vi "Battery mcc.vi"() -> ()   [LabVIEW 2021]
panel:
  in  "stop":bool
  out "length":i32
  in  "Array":dbl[](array[numeric])
  out "String":string
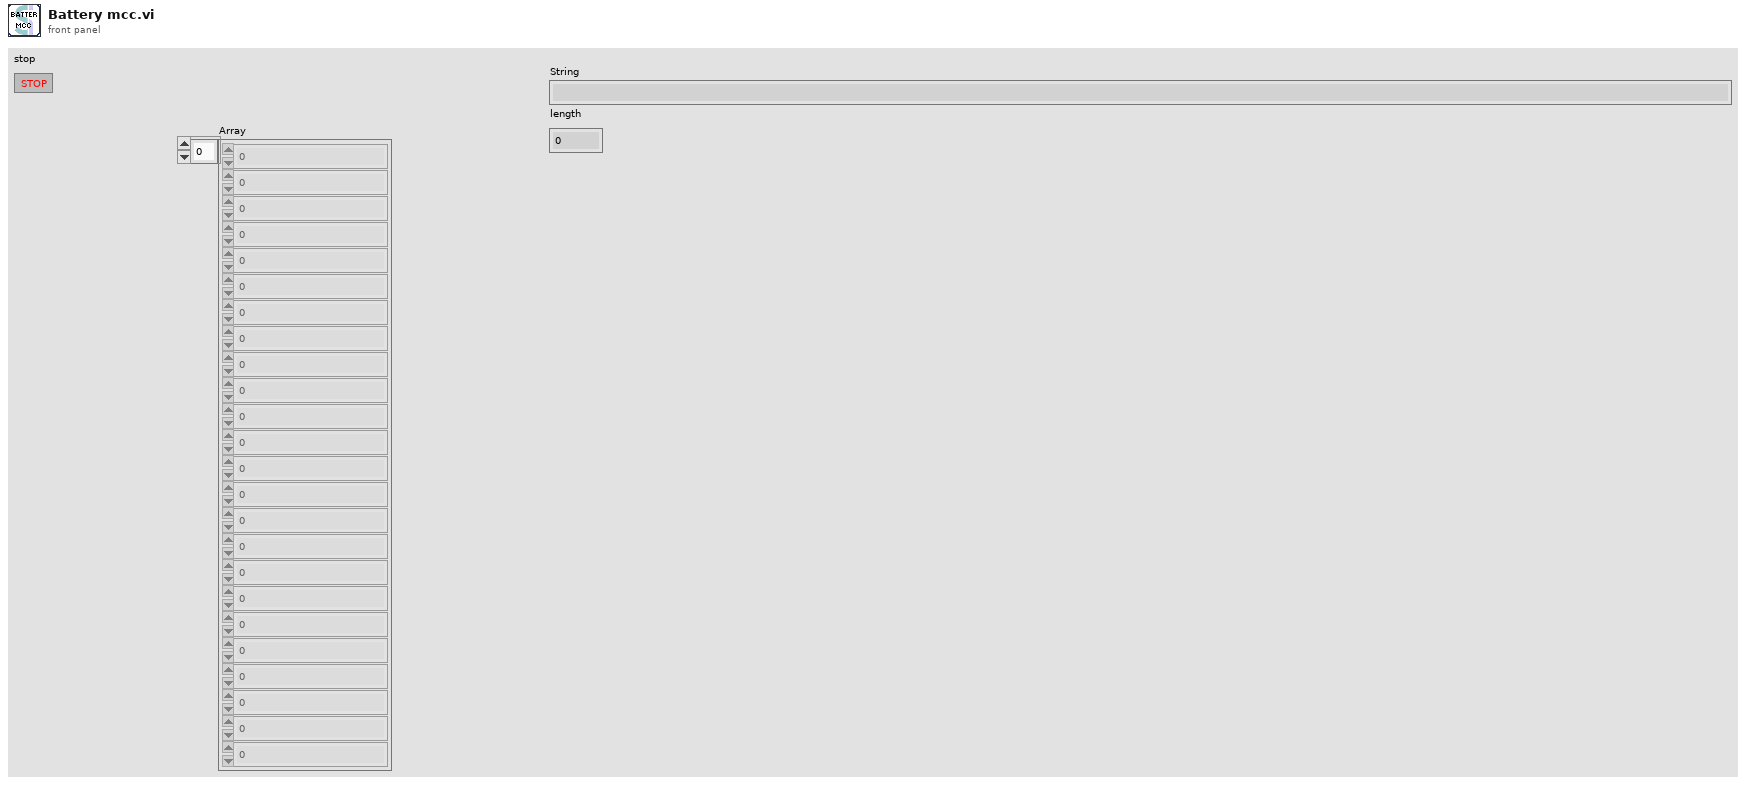
[diagram p1: front panel]
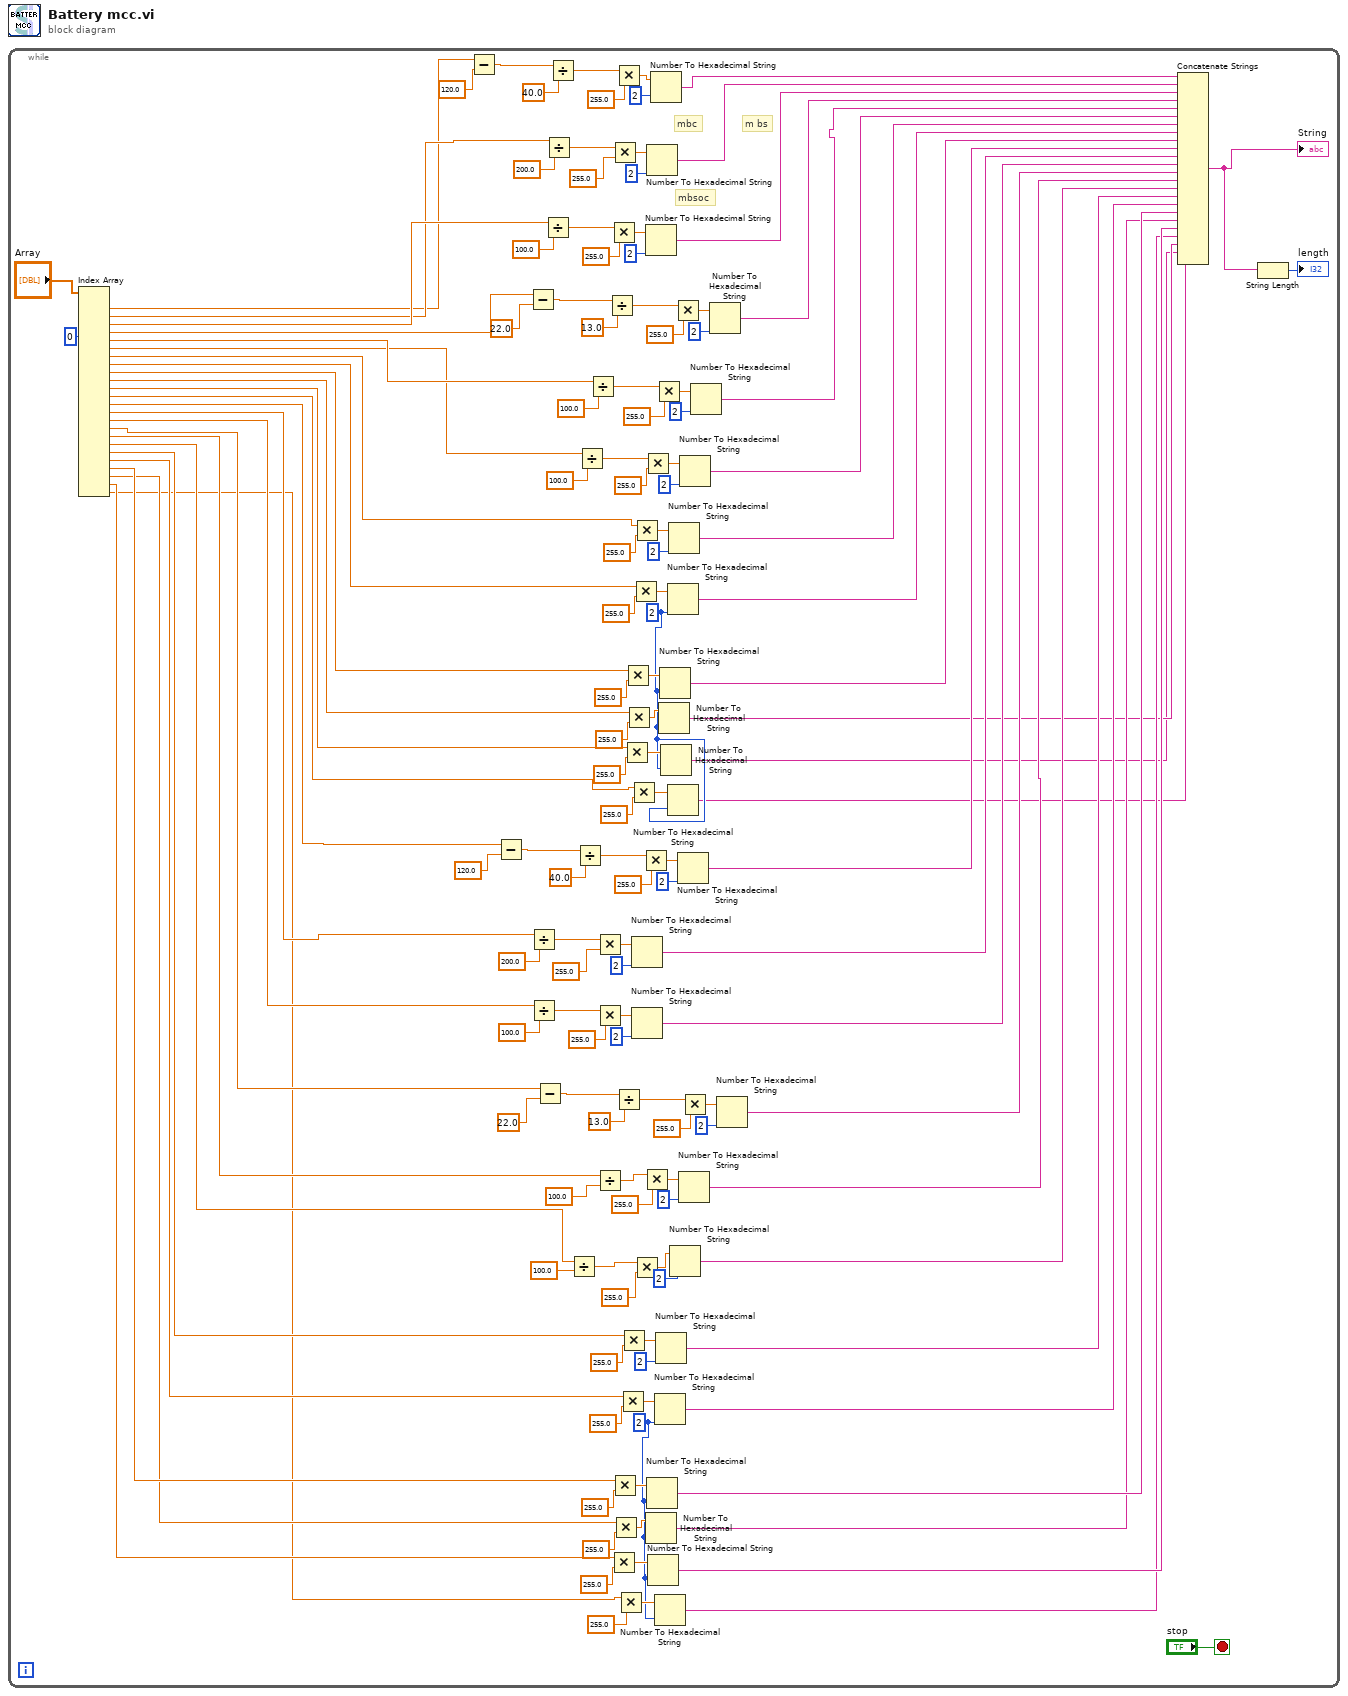
[diagram p0: block diagram]
diagram:
  # "m bs"
  n1 = while {
    stop <- "stop" stop-if-true
    w9 = i16 2 ("width (-)")
    w42 = i16 2 ("width (-)")
    # "mbsoc"
    # "mbc"
    n2 = Index Array(array="Array", index #1=0 ("index")) -> (element #1=w146:dbl, element #2=w147:dbl, element #3=w148:dbl, element #4=w91:dbl, element #5=w90:dbl, element #6=w89:dbl, element #7=w78:dbl, element #8=w77:dbl, element #9=w76:dbl, element #10=w68:dbl, element #11=w67:dbl, element #12=w40:dbl, element #13=w39:dbl, element #14=w38:dbl, element #15=w25:dbl, element #16=w24:dbl, element #17=w23:dbl, element #18=w22:dbl, element #19=w21:dbl, element #20=w20:dbl, element #21=w19:dbl, element #22=w18:dbl, element #23=w17:dbl, element #24=w15:dbl)  [unwired: 23 in]
    n3 = Subtract(x=w146, y=120.0) -> (x-y=w121:dbl)
    n4 = Subtract(x=w39, y=120.0) -> (x-y=w114:dbl)
    n5 = Subtract(x=w91, y=22.0) -> (x-y=w109:dbl)
    n6 = Divide(x=w38, y=200.0) -> (x/y=w113:dbl)
    n7 = Divide(x=w25, y=100.0) -> (x/y=w111:dbl)
    n8 = Subtract(x=w24, y=22.0) -> (x-y=w54:dbl)
    n9 = Divide(x=w148, y=100.0) -> (x/y=w118:dbl)
    n10 = Divide(x=w147, y=200.0) -> (x/y=w120:dbl)
    n11 = Divide(x=w121, y=40.0) -> (x/y=w123:dbl)
    n12 = Divide(x=w22, y=100.0) -> (x/y=w60:dbl)
    n13 = Divide(x=w114, y=40.0) -> (x/y=w116:dbl)
    n14 = Divide(x=w89, y=100.0) -> (x/y=w103:dbl)
    n15 = Divide(x=w90, y=100.0) -> (x/y=w105:dbl)
    n16 = Multiply(x=w113, y=255.0) -> (x*y=w112:dbl)
    n17 = Multiply(x=w111, y=255.0) -> (x*y=w110:dbl)
    n18 = Divide(x=w23, y=100.0) -> (x/y=w58:dbl)
    n19 = Divide(x=w109, y=13.0) -> (x/y=w107:dbl)
    n20 = Multiply(x=w118, y=255.0) -> (x*y=w117:dbl)
    n21 = Multiply(x=w17, y=255.0) -> (x*y=w36:dbl)
    n22 = Multiply(x=w120, y=255.0) -> (x*y=w119:dbl)
    n23 = Multiply(x=w19, y=255.0) -> (x*y=w31:dbl)
    n24 = Multiply(x=w18, y=255.0) -> (x*y=w34:dbl)
    n25 = Multiply(x=w123, y=255.0) -> (x*y=w122:dbl)
    n26 = Divide(x=w54, y=13.0) -> (x/y=w56:dbl)
    n27 = Multiply(x=w15, y=255.0) -> (x*y=w37:dbl)
    n28 = Multiply(x=w20, y=255.0) -> (x*y=w30:dbl)
    n29 = Multiply(x=w21, y=255.0) -> (x*y=w27:dbl)
    n30 = Multiply(x=w67, y=255.0) -> (x*y=w69:dbl)
    n31 = Multiply(x=w76, y=255.0) -> (x*y=w80:dbl)
    n32 = Multiply(x=w68, y=255.0) -> (x*y=w71:dbl)
    n33 = Multiply(x=w40, y=255.0) -> (x*y=w41:dbl)
    n34 = Multiply(x=w77, y=255.0) -> (x*y=w81:dbl)
    n35 = Multiply(x=w78, y=255.0) -> (x*y=w84:dbl)
    n36 = Number To Hexadecimal String(1:i16 2 ("width (-)"), 2:w112) -> (0:w65:string)
    n37 = Number To Hexadecimal String(1:i16 2 ("width (-)"), 2:w110) -> (0:w64:string)
    n38 = Multiply(x=w60, y=255.0) -> (x*y=w59:dbl)
    n39 = Multiply(x=w116, y=255.0) -> (x*y=w115:dbl)
    n40 = Multiply(x=w58, y=255.0) -> (x*y=w57:dbl)
    n41 = Multiply(x=w103, y=255.0) -> (x*y=w104:dbl)
    n42 = Number To Hexadecimal String(1:i16 2 ("width (-)"), 2:w117) -> (0:w92:string)
    n43 = Number To Hexadecimal String(1:w9, 2:w34) -> (0:w11:string)
    n44 = Number To Hexadecimal String(1:i16 2 ("width (-)"), 2:w119) -> (0:w93:string)
    n45 = Number To Hexadecimal String(1:w9, 2:w31) -> (0:w12:string)
    n46 = Number To Hexadecimal String(1:w9, 2:w36) -> (0:w10:string)
    n47 = Number To Hexadecimal String(1:i16 2 ("width (-)"), 2:w122) -> (0:w2:string)
    n48 = Multiply(x=w105, y=255.0) -> (x*y=w106:dbl)
    n49 = Number To Hexadecimal String(1:w9, 2:w30) -> (0:w13:string)
    n50 = Number To Hexadecimal String(1:w9, 2:w37) -> (0:w8:string)
    n51 = Number To Hexadecimal String(1:i16 2 ("width (-)"), 2:w27) -> (0:w14:string)
    n52 = Number To Hexadecimal String(1:w42, 2:w71) -> (0:w6:string)
    n53 = Number To Hexadecimal String(1:w42, 2:w80) -> (0:w73:string)
    n54 = Number To Hexadecimal String(1:w42, 2:w69) -> (0:w5:string)
    n55 = Number To Hexadecimal String(1:w42, 2:w81) -> (0:w74:string)
    n56 = Number To Hexadecimal String(1:w42, 2:w41) -> (0:w4:string)
    n57 = Number To Hexadecimal String(1:i16 2 ("width (-)"), 2:w84) -> (0:w75:string)
    n58 = Number To Hexadecimal String(1:i16 2 ("width (-)"), 2:w59) -> (0:w44:string)
    n59 = Multiply(x=w107, y=255.0) -> (x*y=w108:dbl)
    n60 = Number To Hexadecimal String(1:i16 2 ("width (-)"), 2:w115) -> (0:w66:string)
    n61 = Number To Hexadecimal String(1:i16 2 ("width (-)"), 2:w57) -> (0:w45:string)
    n62 = Number To Hexadecimal String(1:i16 2 ("width (-)"), 2:w104) -> (0:w86:string)
    n63 = Multiply(x=w56, y=255.0) -> (x*y=w55:dbl)
    n64 = Number To Hexadecimal String(1:i16 2 ("width (-)"), 2:w106) -> (0:w87:string)
    n65 = Number To Hexadecimal String(1:i16 2 ("width (-)"), 2:w108) -> (0:w88:string)
    n66 = Number To Hexadecimal String(1:i16 2 ("width (-)"), 2:w55) -> (0:w46:string)
    n67 = Concatenate Strings(w2, w93, w92, w88, w87, w86, w75, w74, w73, w66, w65, w64, w46, w45, w44, w14, w13, w12, w11, w10, w8, w6, w5, w4) -> (w7:string)
    "String" <- w7
    n68 = String Length(string=w7) -> (length=→"length":i32)
  }
